vi "CAN.vi"() -> ()   [LabVIEW 2019]
panel:
  in  "CAN_ID":T1={"LEFT_MASTER_DRIVE"=4, "RIGHT_FRONT_DRIVE"=1, "RIGHT_MASTER_DRIVE"=5, "RIGHT_REAR_DRIVE"=2, "TURRET"=22, "SHOOTER SLAVE"=24, "SHOOTER"=21, "HOPPER"=15, "LEFT_REAR_DRIVE"=3, "LEFT_FRONT_DRIVE"=6, "INTAKE"=11, "INDEXER"=13, "CLIMBER ARM"=0, "CLIMBER WINCH"=0, "SHOOTER ANGLE"=23, "AGITATOR"=14, "AGITATOR OLD"=12}
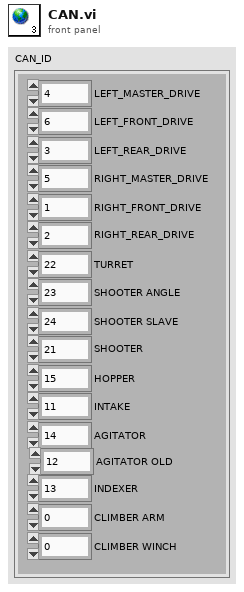
[diagram p1: front panel]
types:
  T1 = cluster{"LEFT_MASTER_DRIVE":u8, "RIGHT_FRONT_DRIVE":u8, "RIGHT_MASTER_DRIVE":u8, "RIGHT_REAR_DRIVE":u8, "TURRET":u8, "SHOOTER SLAVE":u8, "SHOOTER":u8, "HOPPER":u8, "LEFT_REAR_DRIVE":u8, "LEFT_FRONT_DRIVE":u8, "INTAKE":u8, "INDEXER":u8, "CLIMBER ARM":u8, "CLIMBER WINCH":u8, "SHOOTER ANGLE":u8, "AGITATOR":u8, "AGITATOR OLD":u8}
diagram:
